vi "FrontPanel Part2.vi"() -> ()   [LabVIEW 2019]
panel:
  out "m":dbl
  out "n":dbl
  in  "Y2":dbl
  in  "Y1":dbl
  in  "X2":dbl
  in  "X1":dbl
  out "Termòmetre 2":dbl
  in  "Temp. Màxima":i32
  in  "Temp Mínima":i32
  out "Termòmetre digital":dbl
  out "Termòmetre 1":dbl(slide) scale=-40.0..80.0
  in  "stop":bool
  # "SubVI Recta"
  # "y ="
  # "· x   +"
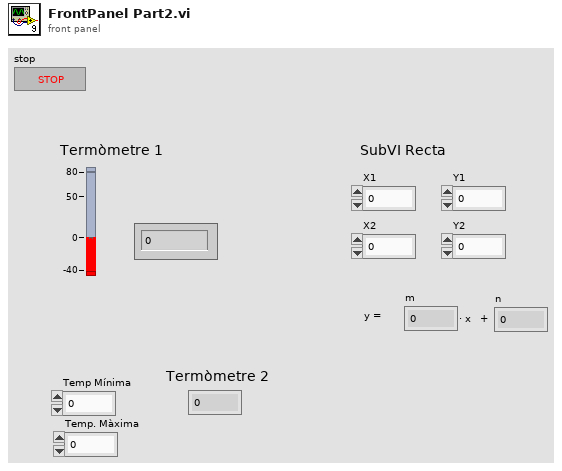
[diagram p1: front panel]
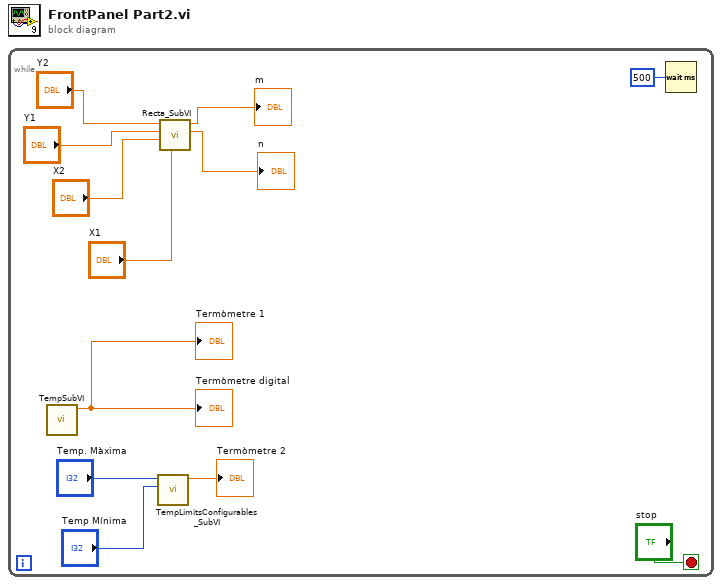
[diagram p0: block diagram]
diagram:
  n1 = while {
    stop <- "stop" stop-if-true
    n2 = call "TempSubVI.vi"() -> ("temp"=→"Termòmetre 1" →"Termòmetre digital":dbl)  [unwired: 11 in]
    n3 = call "TempLimitsConfigurables_SubVI.vi"("TempMin"="Temp Mínima", "TempMax"="Temp. Màxima") -> ("RandomTemp"=→"Termòmetre 2":dbl)  [unwired: 9 in]
    n4 = call "Recta_SubVI.vi"("X1"="X1", "X2"="X2", "Y1"="Y1", "Y2"="Y2") -> ("n"=→"n":dbl, "m"=→"m":dbl)  [unwired: 6 in]
    n5 = Wait (ms)(milliseconds to wait=500) -> ()  [unwired: 1 out]
  }
